vi "第三題.vi"() -> ()   [LabVIEW 2019]
panel:
  in  "stop":bool
  in  "登出":bool
  in  "選手名單":i32[](listbox)=[1, 3, 5]
  in  "比賽選手":i32[](listbox)
  in  "登錄":bool
  # "兩邊名單都可複選。按下登錄後，「選手名單」中的人會移到「比賽選手」中。若按下「登出」則剛好相反。"
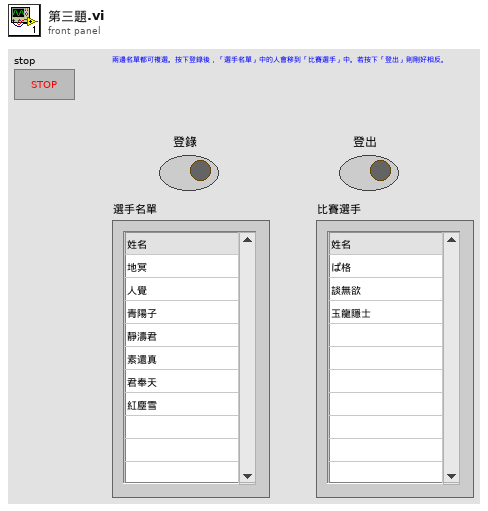
[diagram p1: front panel]
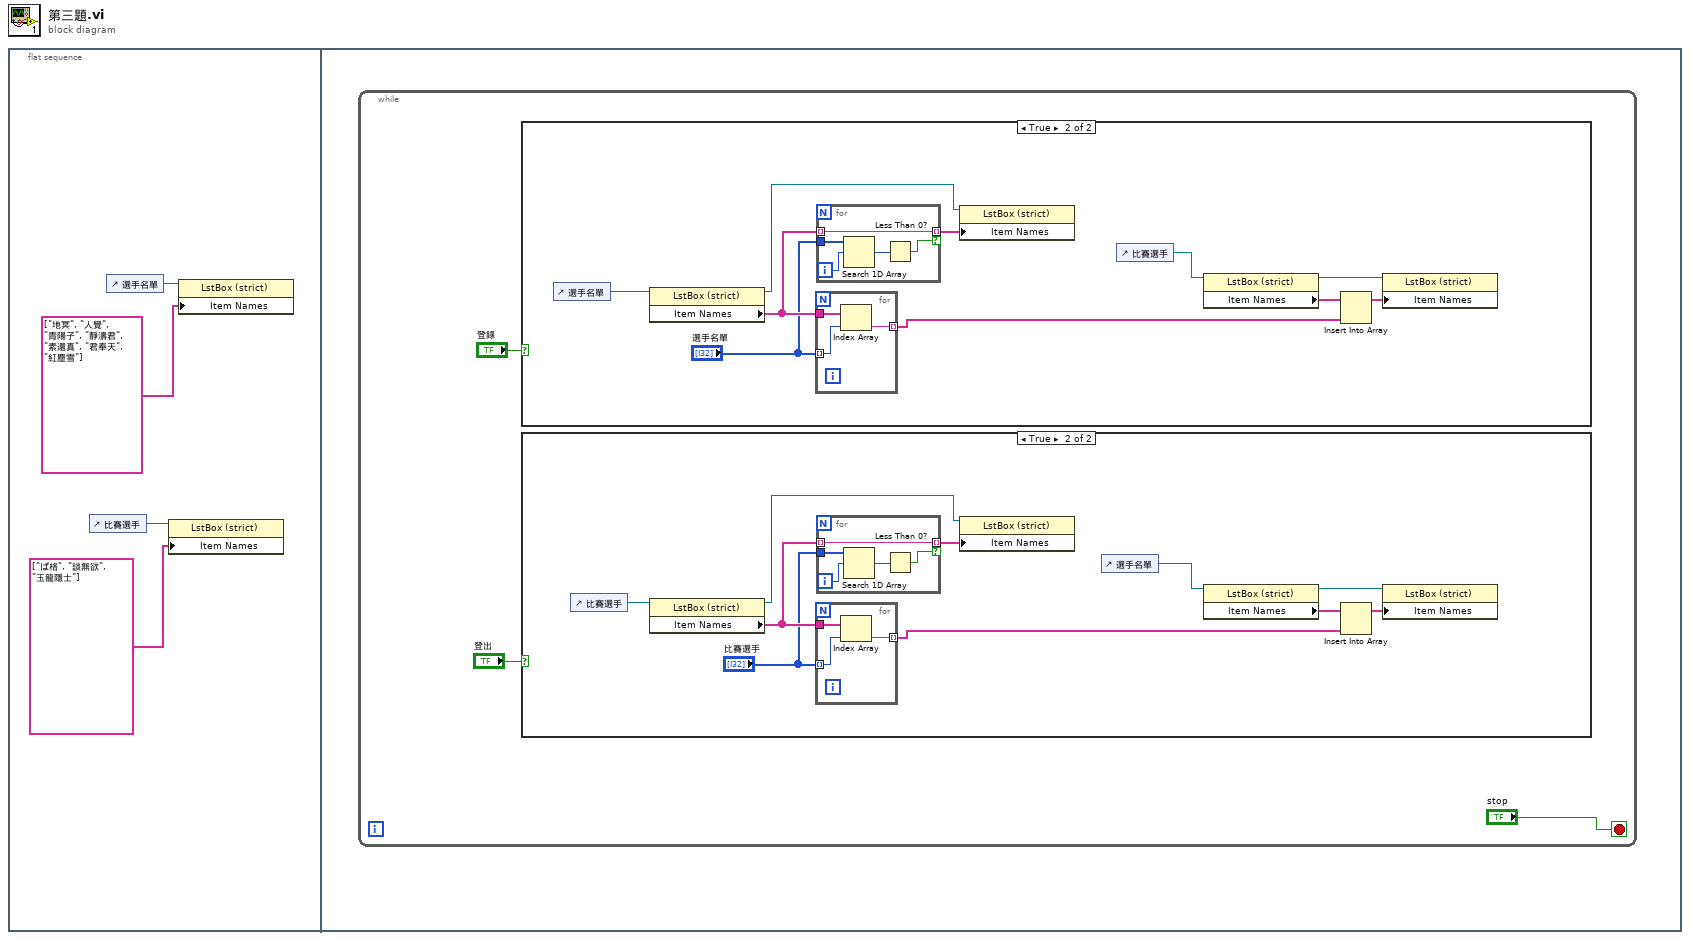
[diagram p0: block diagram]
diagram:
  n1 = flat-sequence {
    frame #0 {
      n2 = control-ref of="比賽選手"() -> (w3:refnum<vi>)
      n3 = control-ref of="選手名單"() -> (w4:refnum<vi>)
      n4 = property on="Property Node" class="LstBox (strict)"(reference=w3, "Item Names"=string[] ["ぱ格", "談無欲", "玉龍隱士"] ("Item Names 2")) -> ()  [unwired: 1 in, 2 out]
      n5 = property on="Property Node" class="LstBox (strict)"(reference=w4, "Item Names"=string[] ["地冥", "人覺", "青陽子", "靜濤君", "素還真", "君奉天", "紅塵雪"]) -> ()  [unwired: 1 in, 2 out]
    }
    frame #1 {
      n6 = while {
        stop <- "stop" stop-if-true
        n7 = case shown="True" "登錄" {
          frame False {
          }
          frame True {
            n8 = control-ref of="選手名單"() -> (w32:refnum<vi>)
            n9 = property on="Property Node" class="LstBox (strict)"(reference=w32) -> (reference out=w26:refnum<vi>, "Item Names"=w29:string[])  [unwired: 1 in, 1 out]
            n10 = for {
              tunnel: w29 -> [w43]
              tunnel: "選手名單" -> [w42] mode=indexing
              tunnel: [w41] -> w34 mode=indexing
              n11 = Index Array(array=w43, index=w42) -> (element=w41:string)
            }
            n12 = for {
              tunnel: w29 -> [w37] mode=indexing
              tunnel: "選手名單" -> [w40]
              tunnel: [w37] -> w27 mode=indexing if=w36
              i -> [w39]
              n13 = Search 1D Array(1D array=w40, element=w39) -> (index of element=w38:i32)  [unwired: 1 in]
              n14 = Less Than 0?(x=w38) -> (x < 0?=w36:bool)
            }
            n15 = property on="Property Node" class="LstBox (strict)"(reference=w26, "Item Names"=w27) -> ()  [unwired: 1 in, 2 out]
            n16 = control-ref of="比賽選手"() -> (w31:refnum<vi>)
            n17 = property on="Property Node" class="LstBox (strict)"(reference=w31) -> (reference out=w30:refnum<vi>, "Item Names"=w35:string[])  [unwired: 1 in, 1 out]
            n18 = Insert Into Array(array=w35, new element=w34) -> (w33:string[])  [unwired: 1 in]
            n19 = property on="Property Node" class="LstBox (strict)"(reference=w30, "Item Names"=w33) -> ()  [unwired: 1 in, 2 out]
          }
        }
        n20 = case shown="True" "登出" {
          frame False {
          }
          frame True {
            n21 = control-ref of="比賽選手"() -> (w9:refnum<vi>)
            n22 = property on="Property Node" class="LstBox (strict)"(reference=w9) -> (reference out=w11:refnum<vi>, "Item Names"=w13:string[])  [unwired: 1 in, 1 out]
            n23 = for {
              tunnel: w13 -> [w25]
              tunnel: "比賽選手" -> [w24] mode=indexing
              tunnel: [w23] -> w16 mode=indexing
              n24 = Index Array(array=w25, index=w24) -> (element=w23:string)
            }
            n25 = for {
              tunnel: w13 -> [w19] mode=indexing
              tunnel: "比賽選手" -> [w22]
              tunnel: [w19] -> w12 mode=indexing if=w18
              i -> [w21]
              n26 = Search 1D Array(1D array=w22, element=w21) -> (index of element=w20:i32)  [unwired: 1 in]
              n27 = Less Than 0?(x=w20) -> (x < 0?=w18:bool)
            }
            n28 = property on="Property Node" class="LstBox (strict)"(reference=w11, "Item Names"=w12) -> ()  [unwired: 1 in, 2 out]
            n29 = control-ref of="選手名單"() -> (w8:refnum<vi>)
            n30 = property on="Property Node" class="LstBox (strict)"(reference=w8) -> (reference out=w14:refnum<vi>, "Item Names"=w17:string[])  [unwired: 1 in, 1 out]
            n31 = Insert Into Array(array=w17, new element=w16) -> (w15:string[])  [unwired: 1 in]
            n32 = property on="Property Node" class="LstBox (strict)"(reference=w14, "Item Names"=w15) -> ()  [unwired: 1 in, 2 out]
          }
        }
      }
    }
  }
